vi "Write Settings_All.vi"(8 "error in (no error)":errorcluster, 10 "Settings_All":T1, 11 "Analog-Output in":refnum<class "Analog-Output.lvclass">) -> (0 "error out":errorcluster, 3 "Analog-Output out":refnum<class "Analog-Output.lvclass">)   [LabVIEW 2019, in "Analog-Output.lvlib" / "Analog-Output.lvclass"]
uses:
  Library/Analog-Output.lvclass
  Custom Controls/Settings.ctl
  Library/Analog-Output.lvclass/Analog-Output.ctl
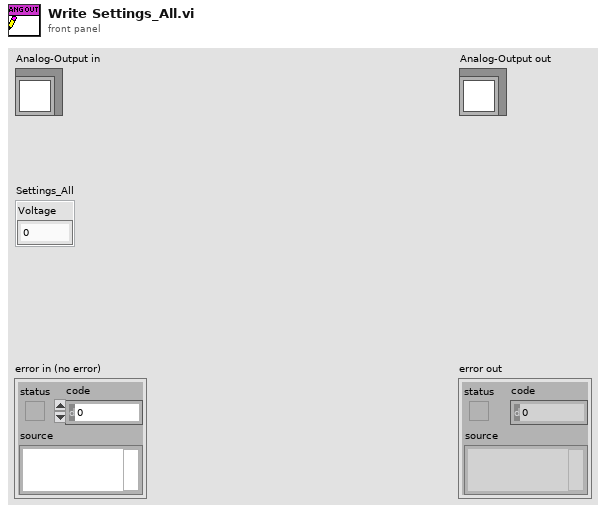
[diagram p1: front panel]
types:
  T1 = typedef "Analog-Output.lvlib/Analog-Output.lvclass/Settings.ctl" = cluster{"Voltage":dbl}
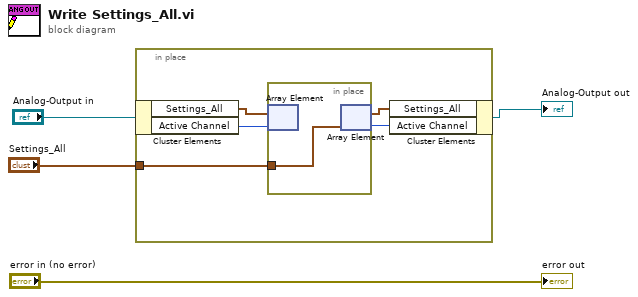
[diagram p0: block diagram]
diagram:
  n1 = in-place {
    in-place-border: "Settings_All" -> [w7]
    n2 = in-place-cluster #1("Analog-Output in") -> ("Settings_All"=w9:T1[], "Active Channel"=w8:u32)
    n3 = in-place {
      in-place-border: w7 -> [w10]
      n4 = in-place-array #2(w9, w8) -> ()  [unwired: 1 out]
      n5 = in-place-array #2(w10) -> (w6:T1[], w5:i32)
    }
    n6 = in-place-cluster #1("Settings_All"=w6, "Active Channel"=w5) -> (→"Analog-Output out":refnum<class "Analog-Output.lvclass">)
  }
  "error out" <- "error in (no error)"
